vi "generate_ht3_header.vi"(4 "nRecords":u64, 6 "SyncRate":i32, 9 "MeasurementMode":i32, 10 "acq_time":i32, 11 "Notes":string) -> (3 "ht3_v2_header":T1={"Ident"=[], "FormatVersion"=[], "CreatorName"=[], "CreatorVersion"=[], "FileTime"=[], "CRLF"=[], "Comment"=[], "NumberOfCurves"=0, "BitsPerRecord"=0, "ActiveCurve"=0, "MeasurementMode"=0, "SubMode"=0, "Binning"=0, "Resolution"=0.0, "Offset"=0, "Tacq"=0, "StopAt"=0, "StoponOvfl"=0, "Restart"=0, "DispLinLog"=0, "DispTimeAxisFrom"=0, "DisplTimeAxisTo"=0, "DispCountAxisFrom"=0, "DispCountAxisTo"=0, "DispCurveMapTo(8)"=[], "DispCurveShow(8)"=[], "ParamStart(3)"=[], "ParamStep(3)"=[], "ParamEnd(3)"=[], "RepeatMode"=0, "RepeatsPerCurve"=0, "Repobjime"=0, "RepeatWaiobjime"=0, "ScriptName"=[], "HardwareIdent"=[], "HardwarePartNo"=[], "HardwareSerial"=0, "nModulesPresent"=1, "ModelCode(10)"=[], "VersionCode(10)"=[], "BaseResolution"=0.0, "inputsEnabled"=0, "InpChansPresent"=8, "RefClockSource"=0, "ExtDevices"=0, "MarkerSeobjings"=0, "SyncDivider"=0, "SyncCFDLevel"=0, "SyncCFDZeroCross"=0, "SyncOffset"=0, "InputModuleIndex(8)"=[], "InputCFDLevel(8)"=[], "InputCFDZeroCross(8)"=[], "InputOffset(8)"=[], "InputRate(8)"=[], "SyncRate"=0, "StopAfter"=0, "StopReason"=0, "ImgHdrSize"=0, "nRecords"=0, "ImgHdr(1)"=[]})   [LabVIEW 2015]
uses:
  ht3_v2_header.ctl
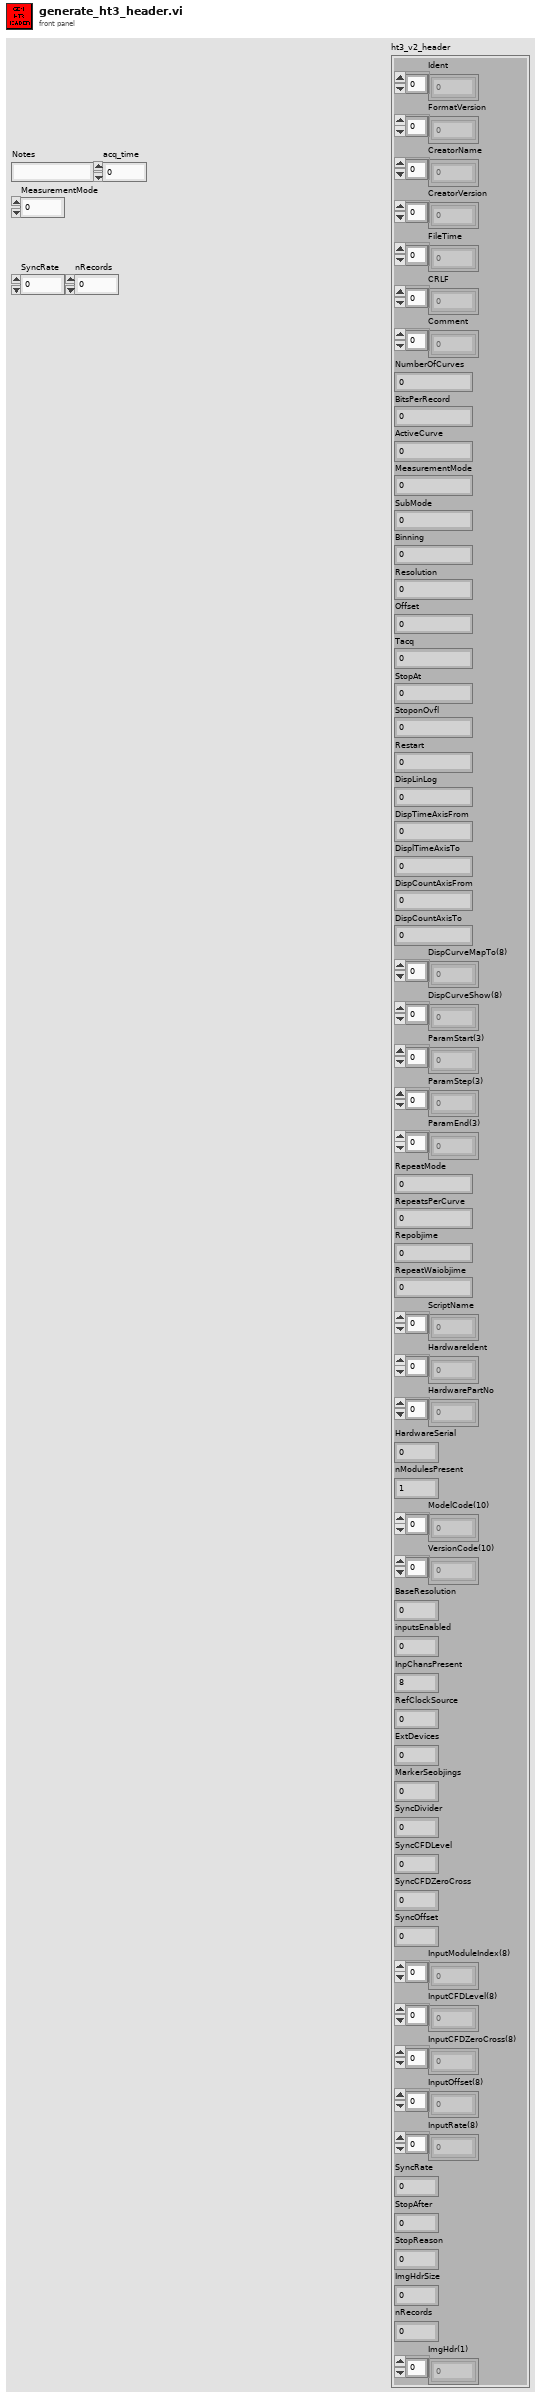
[diagram p1: front panel]
types:
  T1 = typedef "ht3_v2_header.ctl" = cluster{"Ident":u8[], "FormatVersion":u8[], "CreatorName":u8[], "CreatorVersion":u8[], "FileTime":u8[], "CRLF":u8[], "Comment":u8[], "NumberOfCurves":i32, "BitsPerRecord":i32, "ActiveCurve":i32, "MeasurementMode":i32, "SubMode":i32, "Binning":i32, "Resolution":dbl, "Offset":i32, "Tacq":i32, "StopAt":u32, "StoponOvfl":i32, "Restart":i32, "DispLinLog":i32, "DispTimeAxisFrom":i32, "DisplTimeAxisTo":i32, "DispCountAxisFrom":i32, "DispCountAxisTo":i32, "DispCurveMapTo(8)":i32[], "DispCurveShow(8)":i32[], "ParamStart(3)":dbl[], "ParamStep(3)":dbl[], "ParamEnd(3)":dbl[], "RepeatMode":i32, "RepeatsPerCurve":i32, "Repobjime":i32, "RepeatWaiobjime":i32, "ScriptName":u8[], "HardwareIdent":u8[], "HardwarePartNo":u8[], "HardwareSerial":i32, "nModulesPresent":i32, "ModelCode(10)":dbl[], "VersionCode(10)":dbl[], "BaseResolution":dbl, "inputsEnabled":i64, "InpChansPresent":i32, "RefClockSource":i32, "ExtDevices":i32, "MarkerSeobjings":i32, "SyncDivider":i32, "SyncCFDLevel":i32, "SyncCFDZeroCross":i32, "SyncOffset":i32, "InputModuleIndex(8)":i32[], "InputCFDLevel(8)":i32[], "InputCFDZeroCross(8)":i32[], "InputOffset(8)":i32[], "InputRate(8)":i32[], "SyncRate":i32, "StopAfter":i32, "StopReason":i32, "ImgHdrSize":i32, "nRecords":u64, "ImgHdr(1)":i32[]}
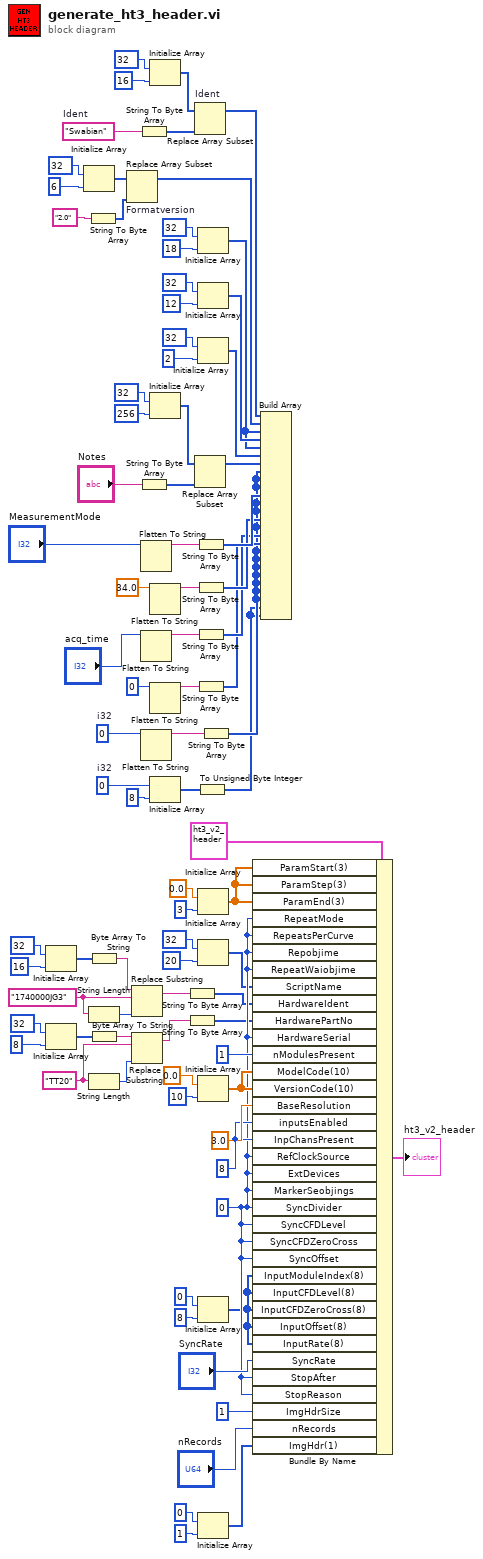
[diagram p0: block diagram]
diagram:
  w4 = 0  # i32
  w19 = 0  # i32
  w55 = i64 8 ("inputsEnabled")
  w41 = "TT20" ("substring (\"\")")
  w43 = "1740000JG3" ("substring (\"\")")
  w51 = 0 ("NumberOfCurves")
  w34 = "Swabian"  # Ident
  n1 = Initialize Array(u8 32, 16 ("dimension size")) -> (w66:u8[])
  n2 = Initialize Array(u8 32, 8 ("dimension size")) -> (w62:u8[])
  n3 = Initialize Array(u8 32, 6 ("dimension size")) -> (w30:u8[])
  n4 = String To Byte Array(string="2.0") -> (unsigned byte array=w31:u8[])
  n5 = Byte Array To String(unsigned byte array=w66) -> (string=w65:string)
  n6 = String Length(string=w43) -> (length=w42:i32)
  n7 = Byte Array To String(unsigned byte array=w62) -> (string=w61:string)
  n8 = String Length(string=w41) -> (length=w40:i32)
  n9 = Replace Array Subset "Formatversion"(array=w30, new element=w31) -> (w24:u8[])  [unwired: 1 in]
  n10 = Replace Substring(2:w42, 4:w43, 5:w65) -> (1:w38:string)  [unwired: 1 in, 1 out]
  n11 = Replace Substring(2:w40, 4:w41, 5:w61) -> (1:w36:string)  [unwired: 1 in, 1 out]
  n12 = String To Byte Array(string=w34) -> (unsigned byte array=w32:u8[])
  n13 = String To Byte Array(string="Notes") -> (unsigned byte array=w28:u8[])
  n14 = Flatten To String(anything="MeasurementMode") -> (data string=w17:string)  [unwired: 3 in, 2 out]
  n15 = Flatten To String(anything="acq_time") -> (data string=w11:string)  [unwired: 3 in, 2 out]
  n16 = Flatten To String(anything=w19) -> (data string=w18:string)  [unwired: 3 in, 2 out]
  n17 = Initialize Array(u8 32, 16 ("dimension size")) -> (w33:u8[])
  n18 = Initialize Array(u8 32, 256 ("dimension size")) -> (w27:u8[])
  n19 = Flatten To String(anything=34.0 ("Resolution")) -> (data string=w14:string)  [unwired: 3 in, 2 out]
  n20 = Flatten To String(anything=u32 0 ("StopAt")) -> (data string=w8:string)  [unwired: 3 in, 2 out]
  n21 = Initialize Array(w4, 8 ("dimension size")) -> (w2:i32[])
  n22 = String To Byte Array(string=w38) -> (unsigned byte array=w37:u8[])
  n23 = String To Byte Array(string=w36) -> (unsigned byte array=w35:u8[])
  n24 = Replace Array Subset "Ident"(array=w33, new element=w32) -> (w25:u8[])  [unwired: 1 in]
  n25 = Replace Array Subset(array=w27, new element=w28) -> (w20:u8[])  [unwired: 1 in]
  n26 = String To Byte Array(string=w17) -> (unsigned byte array=w15:u8[])
  n27 = String To Byte Array(string=w14) -> (unsigned byte array=w12:u8[])
  n28 = String To Byte Array(string=w11) -> (unsigned byte array=w9:u8[])
  n29 = String To Byte Array(string=w8) -> (unsigned byte array=w6:u8[])
  n30 = To Unsigned Byte Integer(number=w2) -> (unsigned 8bit integer=w1:u8[])
  n31 = Initialize Array(u8 32, 18 ("dimension size")) -> (w22:u8[])
  n32 = Initialize Array(u8 32, 12 ("dimension size")) -> (w23:u8[])
  n33 = Initialize Array(u8 32, 2 ("dimension size")) -> (w21:u8[])
  n34 = Initialize Array(0.0 ("element"), 3 ("dimension size")) -> (w71:dbl[])
  n35 = Initialize Array(u8 32, 20 ("dimension size")) -> (w39:u8[])
  n36 = Initialize Array(0.0 ("element"), 10 ("dimension size")) -> (w58:dbl[])
  n37 = Initialize Array(0 ("element"), 8 ("dimension size")) -> (w44:i32[])
  n38 = Initialize Array(0 ("element"), 1 ("dimension size")) -> (w47:i32[])
  n39 = String To Byte Array(string=w18) -> (unsigned byte array=w5:u8[])
  n40 = Bundle By Name(cluster=T1 {"Ident"=[], "FormatVersion"=[], "CreatorName"=[], "CreatorVersion"=[], "FileTime"=[], "CRLF"=[], "Comment"=[], "NumberOfCurves"=0, "BitsPerRecord"=0, "ActiveCurve"=0, "MeasurementMode"=0, "SubMode"=0, "Binning"=0, "Resolution"=0.0, "Offset"=0, "Tacq"=0, "StopAt"=0, "StoponOvfl"=0, "Restart"=0, "DispLinLog"=0, "DispTimeAxisFrom"=0, "DisplTimeAxisTo"=0, "DispCountAxisFrom"=0, "DispCountAxisTo"=0, "DispCurveMapTo(8)"=[], "DispCurveShow(8)"=[], "ParamStart(3)"=[], "ParamStep(3)"=[], "ParamEnd(3)"=[], "RepeatMode"=0, "RepeatsPerCurve"=0, "Repobjime"=0, "RepeatWaiobjime"=0, "ScriptName"=[], "HardwareIdent"=[], "HardwarePartNo"=[], "HardwareSerial"=0, "nModulesPresent"=1, "ModelCode(10)"=[], "VersionCode(10)"=[], "BaseResolution"=0.0, "inputsEnabled"=0, "InpChansPresent"=8, "RefClockSource"=0, "ExtDevices"=0, "MarkerSeobjings"=0, "SyncDivider"=0, "SyncCFDLevel"=0, "SyncCFDZeroCross"=0, "SyncOffset"=0, "InputModuleIndex(8)"=[], "InputCFDLevel(8)"=[], "InputCFDZeroCross(8)"=[], "InputOffset(8)"=[], "InputRate(8)"=[], "SyncRate"=0, "StopAfter"=0, "StopReason"=0, "ImgHdrSize"=0, "nRecords"=0, "ImgHdr(1)"=[]} ("Cluster"), "ParamStart(3)"=w71, "ParamStep(3)"=w71, "ParamEnd(3)"=w71, "RepeatMode"=w51, "RepeatsPerCurve"=w51, "Repobjime"=w51, "RepeatWaiobjime"=w51, "ScriptName"=w39, "HardwareIdent"=w37, "HardwarePartNo"=w35, "HardwareSerial"=w51, "nModulesPresent"=1, "ModelCode(10)"=w58, "VersionCode(10)"=w58, "BaseResolution"=3.0, "inputsEnabled"=w55, "InpChansPresent"=w55, "RefClockSource"=w51, "ExtDevices"=w51, "MarkerSeobjings"=w51, "SyncDivider"=w51, "SyncCFDLevel"=w51, "SyncCFDZeroCross"=w51, "SyncOffset"=w51, "InputModuleIndex(8)"=w44, "InputCFDLevel(8)"=w44, "InputCFDZeroCross(8)"=w44, "InputOffset(8)"=w44, "InputRate(8)"=w44, "SyncRate"="SyncRate", "StopAfter"=w51, "StopReason"=w51, "ImgHdrSize"=1, "nRecords"="nRecords", "ImgHdr(1)"=w47) -> (→"ht3_v2_header":T1)
  n41 = Build Array(w25, w24, w22, w23, w22, w21, w20, w5, w5, w5, w15, w5, w5, w12, w5, w9, w6, w5, w5, w5, w5, w5, w5, w5, w1, w1) -> ()  [unwired: 1 out]
